vi "Functions.vi"() -> ()   [LabVIEW 2019]
panel:
  out "Fahrenheit Value":dbl
  out "Fahrenheit":dbl(slide) scale=32.0..212.0
  in  "Celsius":dbl(slide) scale=0.0..100.0
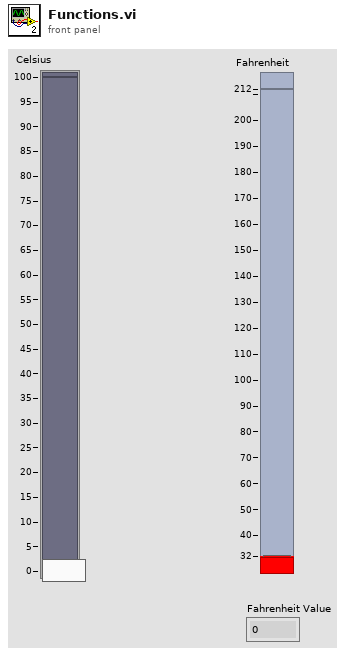
[diagram p1: front panel]
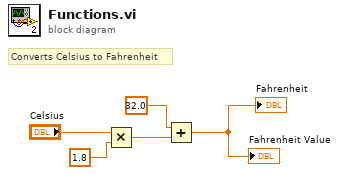
[diagram p0: block diagram]
diagram:
  # "Converts Celsius to Fahrenheit"
  n1 = Multiply(x="Celsius", y=1.8) -> (x*y=w3:dbl)
  n2 = Add(x=32.0, y=w3) -> (x+y=→"Fahrenheit" →"Fahrenheit Value":dbl)
